vi "Read Signal Suffix.vi"(8 "error in (no error)":errorcluster, 11 "IMD_ACP in":refnum<class "IMD_ACP.lvclass">) -> (0 "error out":errorcluster, 2 "Signal Suffix":string, 3 "IMD_ACP out":refnum<class "IMD_ACP.lvclass">)   [LabVIEW 2018, in "SeqAuto Evaluations.lvlib" / "IMD_ACP.lvclass"]
uses:
  IMD_ACP.lvclass
  IMD_ACP.lvclass/IMD_ACP.ctl
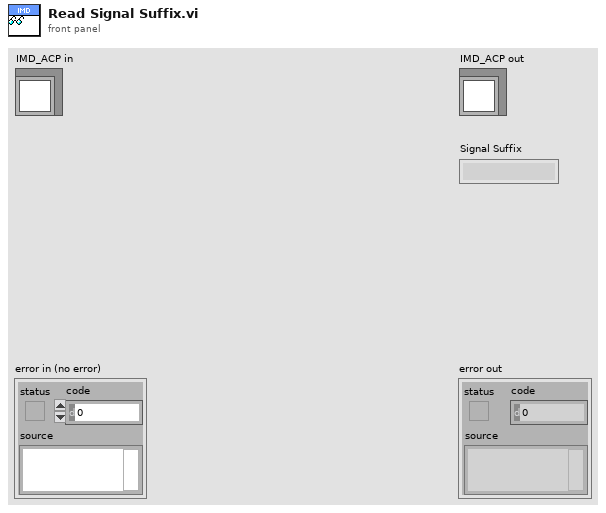
[diagram p1: front panel]
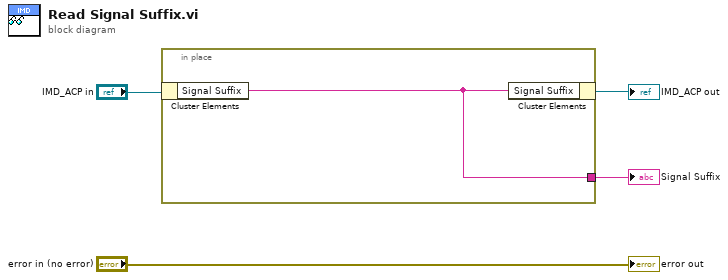
[diagram p0: block diagram]
diagram:
  n1 = in-place {
    in-place-border: [w5] -> w2
    n2 = in-place-cluster #1("IMD_ACP in") -> ("Signal Suffix"=w5:string)
    n3 = in-place-cluster #1("Signal Suffix"=w5) -> (→"IMD_ACP out":refnum<class "IMD_ACP.lvclass">)
  }
  "Signal Suffix" <- w2
  "error out" <- "error in (no error)"
